vi "Get settings chain.vi"(8 "error in (no error)":errorcluster, 11 "MeritFactorBase in":refnum<class "MeritFactor.lvclass">) -> (0 "error out":errorcluster, 1 "class name":string[](array[string]), 2 "settings":variant[](array[variant]), 3 "MeritFactorBase out":refnum<class "MeritFactor.lvclass">)   [LabVIEW 2012, in "MeritFactor.lvclass"]
doc: "Returns an array of variants containing the settings clusters of each class in the inheritance chain (lowest child class first), together with an array of all class names in the inheritance chain.\n\nFor classes without settings cluster, the settings chain contains empty variants."
uses:
  MeritFactor.lvclass
  <vilib>/Distrio/Murmex/Murmex/Murmex.lvclass
  MeritFactor.lvclass/MeritFactor.ctl
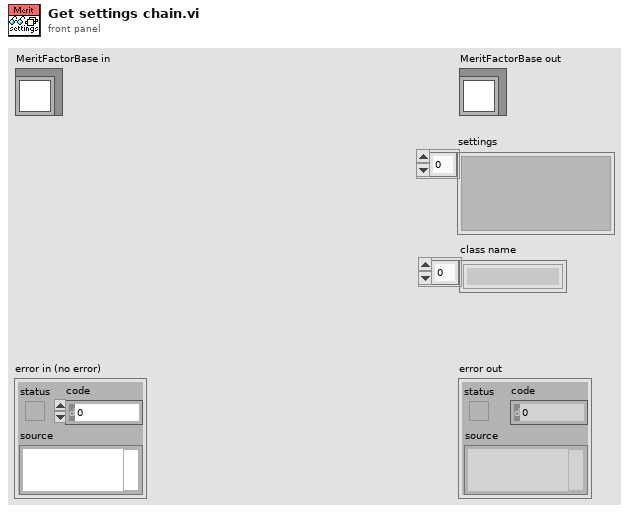
[diagram p1: front panel]
types:
  T1 = typedef "MeritFactor.lvclass/settings cluster.ctl" = cluster{"Brightest bins":i32, "Merit Factor":dbl, "Threshold":sgl}
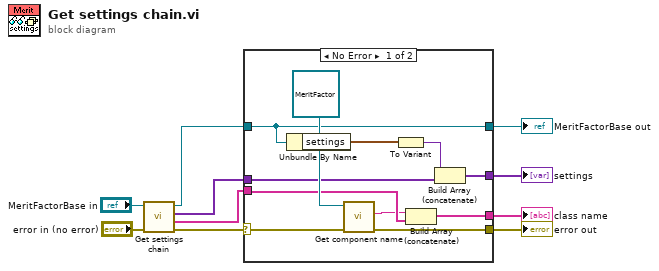
[diagram p0: block diagram]
diagram:
  n1 = call-parent "Get settings chain.vi"("error in (no error)"="error in (no error)", "MurmexBase in"="MeritFactorBase in") -> ("error out"=w8:errorcluster, "class name"=w6:string[], "settings"=w4:variant[], "MurmexBase out"=w3:refnum<class "MeritFactor.lvclass">)  [unwired: 6 in]
  n2 = case shown="No Error" w8 {
    selector: w8 -> [w20 w23]
    tunnel: [w19 w23] -> w7
    tunnel: w6 -> [w18 w22]
    tunnel: [w16 w22] -> w5
    tunnel: w4 -> [w15 w24]
    tunnel: w3 -> [w14 w25]
    tunnel: [w14 w25] -> w2
    tunnel: [w11 w24] -> w1
    frame No Error {
      n3 = Unbundle By Name(w14) -> ("settings"=w13:T1)
      n4 = call <vilib>:"Get component name.vi"("error in (no error)"=w20, "Murmex in"=refnum<class "MeritFactor.lvclass"> refnum ("MeritFactor")) -> ("error out"=w19:errorcluster, "component name"=w17:string)  [unwired: 7 in, 1 out]
      n5 = To Variant(anything=w13) -> (Variant=w12:variant)
      n6 = Build Array (concatenate)(w17, w18) -> (w16:string[])
      n7 = Build Array (concatenate)(w12, w15) -> (w11:variant[])
    }
    frame Error {
    }
  }
  "error out" <- w7
  "MeritFactorBase out" <- w2
  "settings" <- w1
  "class name" <- w5
